vi "Plant_Name_to_CH.vi"(8 "Error In":errorcluster, 10 "Plant Name":string, 11 "Plants_Digital_OP":T1 {"Channel No" items=["7"=7, "11"=11, "12"=12, "13"=13, "15"=15, "16"=16, "18"=18, "29"=29, "32"=32, "33"=33, "35"=35, "36"=36, "37"=37, "38"=38, "40"=40]}) -> (0 "Error Out":errorcluster, 1 "Index":i32, 2 "No":u8, 3 "Channel No":u8)   [LabVIEW 2014, in "TimeBasedProd.lvlib"]
uses:
  TimeBasedProd.lvlib
  TypeDef/Plant_OP_Map.ctl
  TypeDef/Plant_OP_Map_CTR.ctl
  ValveCTRL/TypeDef/CHs_List.ctl
  ValveCTRL/ValveCTRL.lvlib
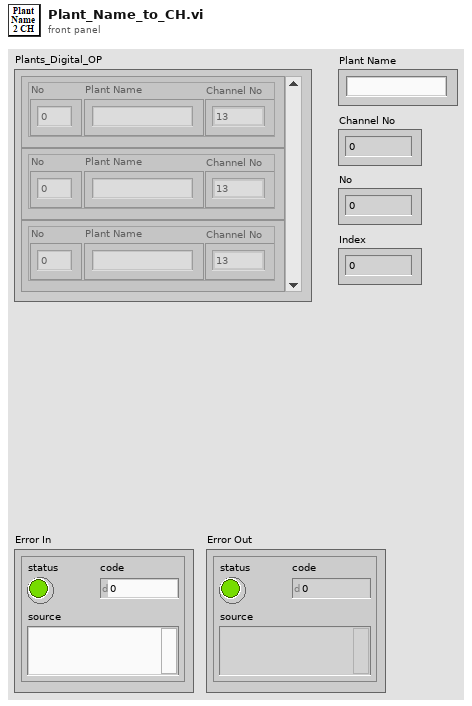
[diagram p1: front panel]
types:
  T1 = typedef "TimeBasedProd.lvlib/Plant_OP_Map.ctl" = T2[]
  T2 = typedef "TimeBasedProd.lvlib/Plant_OP_Map_CTR.ctl" = cluster{"No":u8, "Plant Name":string, "Channel No":T3}
  T3 = typedef "ValveCTRL.lvlib/CHs_List.ctl" = u8
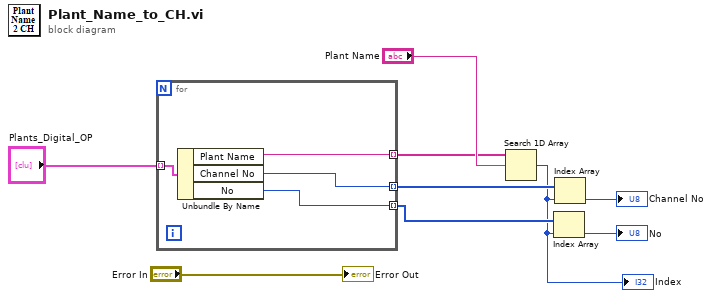
[diagram p0: block diagram]
diagram:
  n1 = for {
    tunnel: "Plants_Digital_OP" -> [w13] mode=indexing
    tunnel: [w12] -> w6 mode=indexing
    tunnel: [w11] -> w5 mode=indexing
    tunnel: [w10] -> w3 mode=indexing
    n2 = Unbundle By Name(w13) -> ("Plant Name"=w12:string, "Channel No"=w11:T3, "No"=w10:u8)
  }
  n3 = Search 1D Array(1D array=w6, element="Plant Name") -> (index of element=w2:i32)  [unwired: 1 in]
  "Index" <- w2
  n4 = Index Array(array=w3, index=w2) -> (element=→"No":u8)
  n5 = Index Array(array=w5, index=w2) -> (element=→"Channel No":T3)
  "Error Out" <- "Error In"
